vi "TestingVI.vi"() -> ()   [LabVIEW 2011]
uses:
  ROV/Vessel.lvclass
  Controller/Controller.lvclass
  Guidance/Guidance.lvclass
  Thrust Allocation/Thrust Allocation().vi
  Thrust Allocation/Thrust Allocation.lvclass
panel:
  out "Observer Names":string[](array[string])
  out "Controller Names":string[](array[string])
  in  "File Path Control":path=path "D:/Espen Tolpinrud/My Documents/LabView/AUR Control System/ROV/Configuration"
  in  "ROV Selector":u16(ring) items=["Minerva", "Neptune"]
  out "Guidance Array":refnum<class "Guidance.lvclass">[](array[class])
  out "Array Controllers":refnum<class "Controller.lvclass">[](array[class])
  out "Vessel Out":refnum<class "Vessel.lvclass">
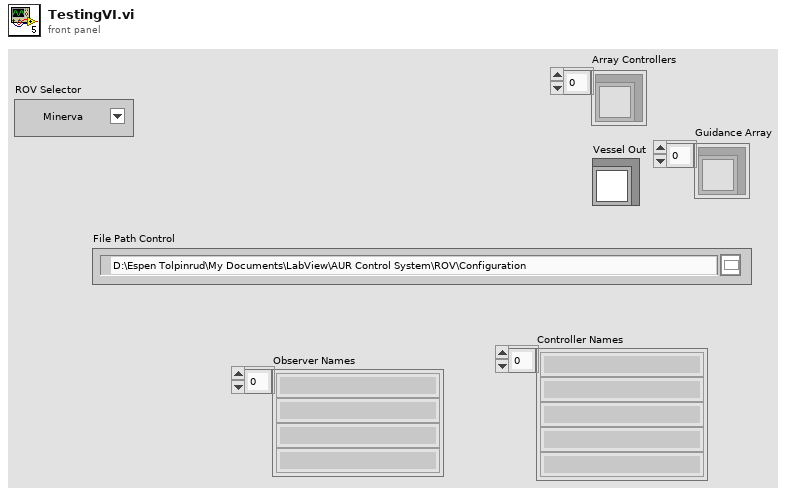
[diagram p1: front panel]
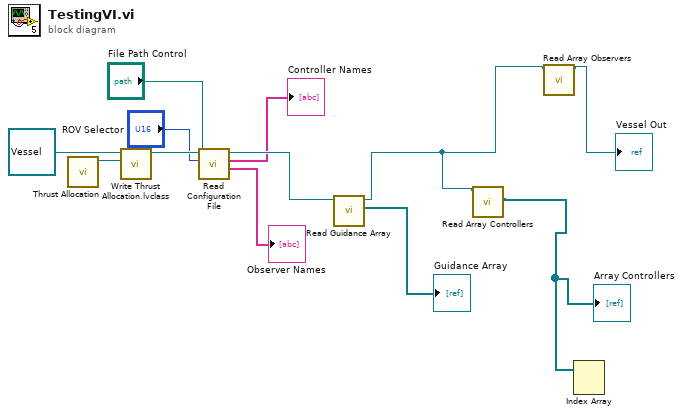
[diagram p0: block diagram]
diagram:
  n1 = call-poly "Thrust Allocation.vi"() -> ("Thrust Allocation Out"=w12:refnum<class "Thrust Allocation.lvclass">)  [unwired: 11 in]
  n2 = call "Write Thrust Allocation.lvclass.vi"("Thrust Allocation.lvclass"=w12, "Vessel in"=refnum<class "Vessel.lvclass"> refnum ("Vessel.lvclass")) -> ("Vessel out"=w10:refnum<class "Vessel.lvclass">)  [unwired: 8 in, 1 out]
  n3 = call "Read Configuration File.vi"("File Path Control"="File Path Control", "ROV Selector"="ROV Selector", "Vessel In"=w10) -> ("Observer Names"=→"Observer Names":string[], "Controller Names"=→"Controller Names":string[], "Vessel Out"=w9:refnum<class "Vessel.lvclass">)  [unwired: 5 in, 1 out]
  n4 = call "Read Guidance Array.vi"("Vessel in"=w9) -> ("Guidance Array"=→"Guidance Array":refnum<class "Guidance.lvclass">[], "Vessel out"=w3:refnum<class "Vessel.lvclass">)  [unwired: 8 in, 1 out]
  n5 = call "Read Array Controllers.vi"("Vessel in"=w3) -> ("Array Controllers"=w7:refnum<class "Controller.lvclass">[])  [unwired: 8 in, 2 out]
  "Array Controllers" <- w7
  n6 = call-dynamic "Read Array Observers.vi"("Vessel in"=w3) -> ("Vessel out"=→"Vessel Out":refnum<class "Vessel.lvclass">)  [unwired: 8 in, 2 out]
  n7 = Index Array(array=w7) -> ()  [unwired: 2 in, 2 out]
